vi "MeasureDistanceInImage.vi"() -> ()   [LabVIEW 2016]
uses:
  <vilib>/vision/NI_Vision_Development_Module.lvlib
  <vilib>/Utility/inputDevices.llb/mouseAcquire.vi
panel:
  in  "Pitch":dbl=75.5
  in  "Npixels":dbl=774.031
  in  "Nstrips":dbl=17.0
  out "Length (um)":dbl=1283.499968605464
  out "Conversion: \n1 pixel to um":dbl=1.6582023200621165
  out "Length (Pixels)":dbl=774.0309810671256
  out "Position 2":cluster{"X2 Value":dbl, "Y2 Value":dbl}={"X2 Value"=1797.893287435456, "Y2 Value"=1434.5183016105418}
  in  "Set Position 2":bool=TRUE
  out "Position 1":cluster{"X1 Value":dbl, "Y1 Value":dbl}={"X1 Value"=2571.9242685025815, "Y1 Value"=1434.5183016105418}
  in  "Set Position 1":bool=TRUE
  out "Analysis Image":T1(plugin-control)
  out "error out":errorcluster
  in  "X coord":dbl(slide)=1797.893287435456 max=2592.0 scale=0.0..3840.0
  in  "Y coord":dbl(slide)=1434.5183016105418 max=1944.0
  out "axis info":T2
  out "Array":T3(array[cluster])
  out "Intensity Histogram":T4(graph)={"Starting Value"=0.0, "Incremental Value"=1.0, "Histogram"=[197, 7029, 132892, 970999, 1117168, 291828, 56433, 20526, 12325, 9713, 7377, 5795, 5651, 5314, 3720, 2616, 1826, 1549, 1730, 1683, 1402, 1473, 1424, 1279, 1558, 1557, 1323, 1503, 1470, 1441, 1598, 1708, 1752, 2278, 2684, 3297, 5038, 7928, 11020, 15856, 18444, 15887, 15408, 15022, 16873, 25059, 31763, 32994, 39559, 44318, 45818, 56557, 59745, 55325, 61336, 58801, 49186, 48315, 39061, 30075, 29526, 26387, 22284, 22031, 20409, 17373, 17024, 16091, 13164, 13088, 12293, 10119, 10289, 9463, 7808, 8013, 7680, 6634, 7304, 7199, 6356, 6959, 6712, 5915, 6605, 6512, 5771, 6500, 6373, 6066, 6669, 6627, 6337, 6938, 7422, 7246, 8047, 8727, 8566, 10407, 11503, 11840, 14142, 16803, 17562, 22809, 26304, 27447, 33496, 37329, 37032, 44436, 46230, 42854, 47790, 47201, 42637, 44791, 43072, 37704, 38373, 35741, 30906, 30613, 28123, 23550, 24512, 22759, 19529, 19195, 18077, 15460, 16338, 15747, 13203, 13914, 13230, 11109, 11903, 10976, 8982, 9154, 8056, 6836, 6374, 5448, 4144, 3761, 2999, 2167, 1811, 1352, 905, 721, 529, 313, 215, 155, 87, 72, 41, 19, 11, 9, 3, 2, 1, 1, 0, 0, 0, 0, 0, 0, 0, 0, 0, 0, 0, 0, 0, 0, 0, 0, 0, 0, 0, 0, 0, 0, 0, 0, 0, 0, 0, 0, 0, 0, 0, 0, 0, 0, 0, 0, 0, 0, 0, 0, 0, 0, 0, 0, 0, 0, 0, 0, 0, 0, 0, 0, 0, 0, 0, 0, 0, 0, 0, 0, 0, 0, 0, 0, 0, 0, 0, 0, 0, 0, 0, 0, 0, 0, 0, 0, 0, 0, 0, 0, 0, 0, 0, 0, 0, 0, 0, 0]}
  in  "Path":path=path "E:/BNL/XYZstage+Camera_CollectedImages/02-06-2017/images/image_00_-53_-30_-1.png"
  # "Measure a distance in an image"
  # "Supply data for calibration calculation"
  # "readoutstrips_2 : 42, 956.746, 75.5\nSzoom1 : 16, 2323, 75.5"
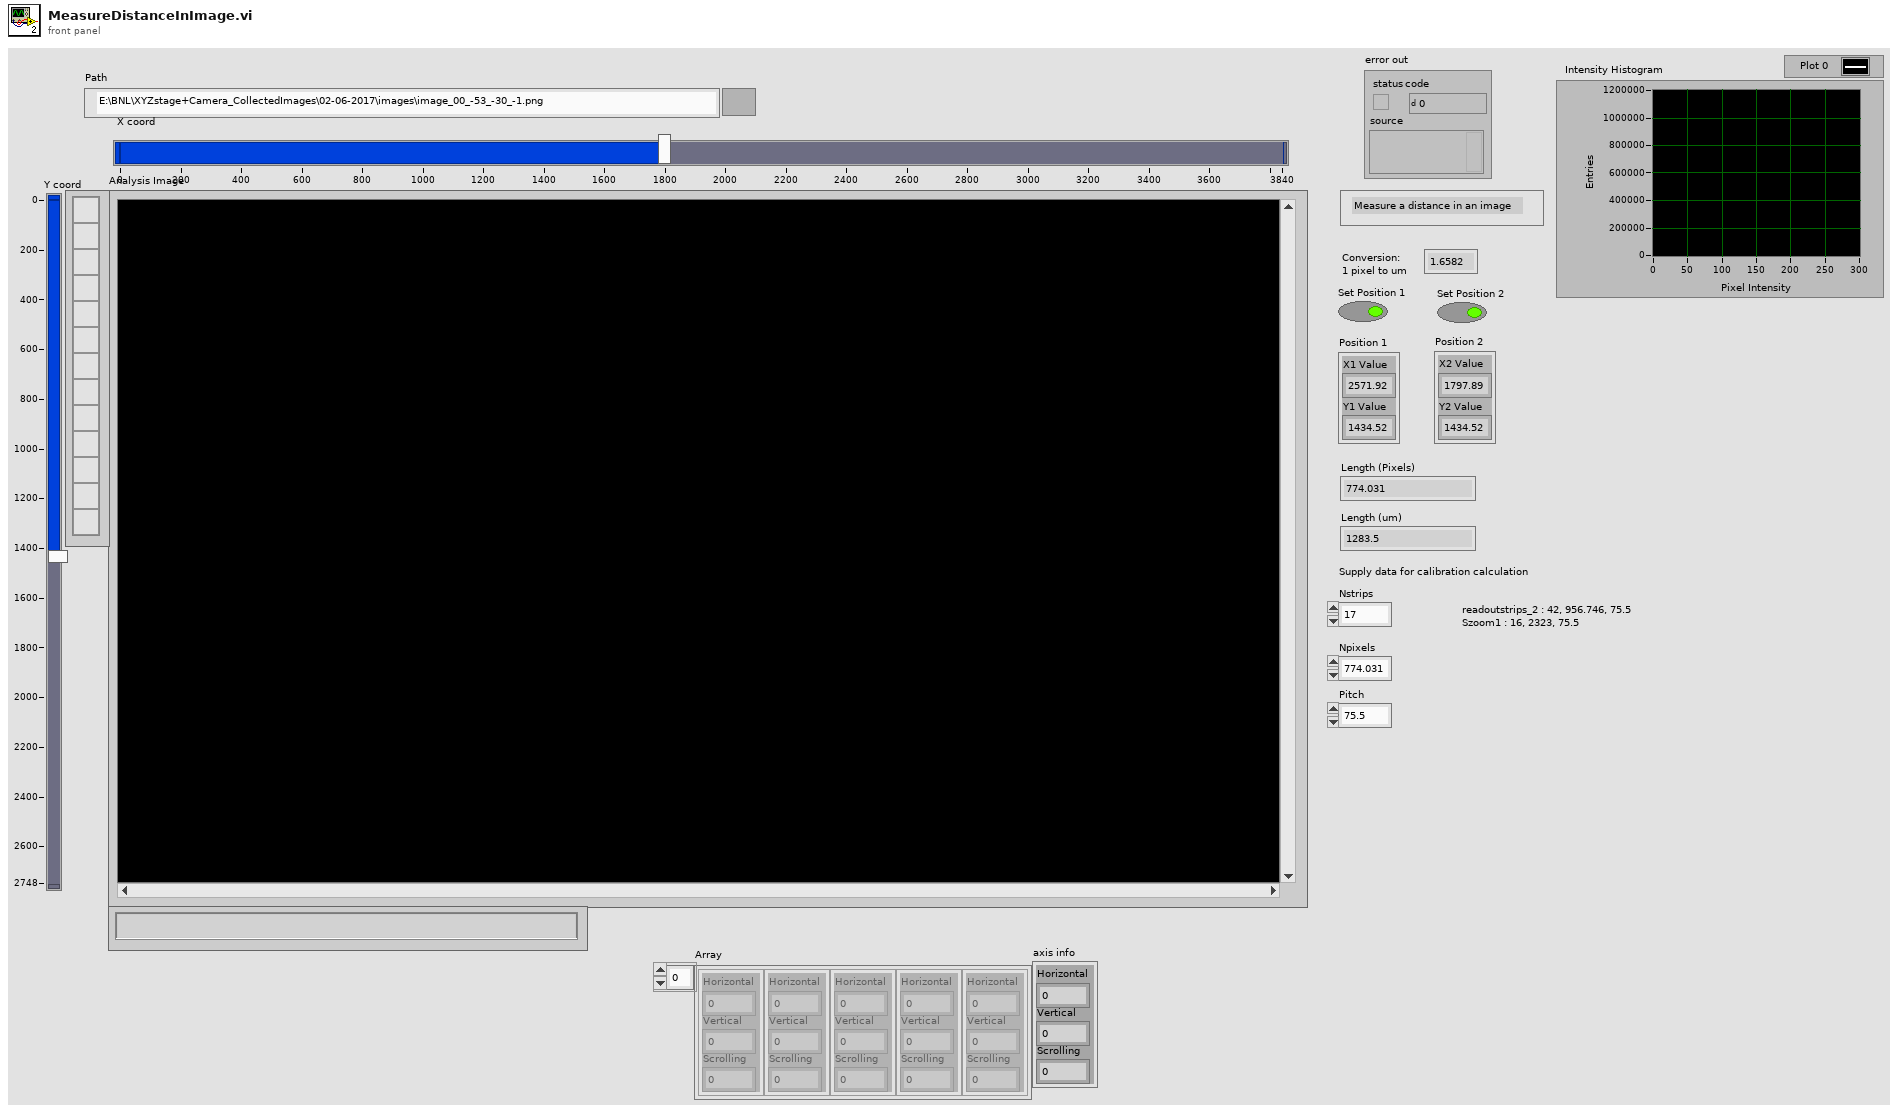
[diagram p1: front panel]
types:
  T1 = typedef "IMAQ Image.ctl" = refnum<image>
  T2 = cluster{"Horizontal":i32, "Vertical":i32, "Scrolling":i32}
  T3 = cluster{"Horizontal":i32, "Vertical":i32, "Scrolling":i32}[]
  T4 = cluster{"Starting Value":sgl, "Incremental Value":sgl, "Histogram":u32[]}
  T5 = cluster{"button 1":bool, "button 2":bool, "button 3":bool, "button 4":bool}
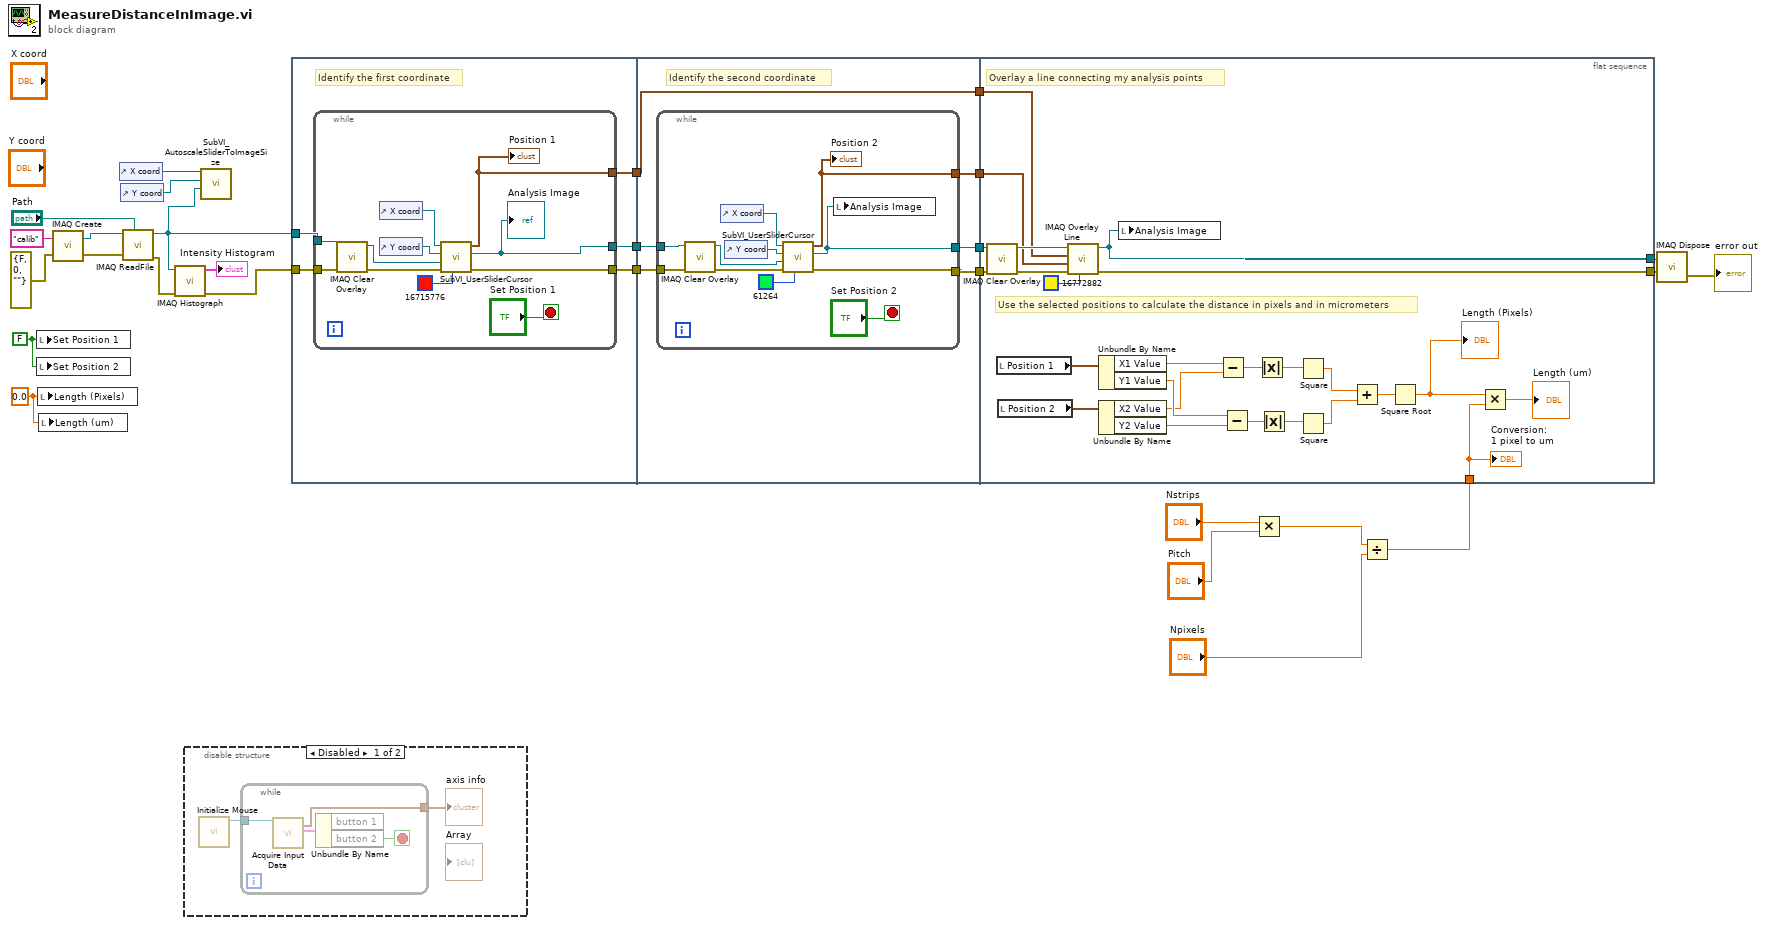
[diagram p0: block diagram]
diagram:
  w6 = 0.0 ("Length (Pixels)")
  w8 = FALSE ("Set Position 1")
  n1 = local write "Set Position 1"(w8) -> ()
  n2 = local write "Set Position 2"(w8) -> ()
  n3 = local write "Length (Pixels)"(w6) -> ()
  n4 = local write "Length (um)"(w6) -> ()
  n5 = call "IMAQ Create"("Image Name"="calib", "error in (no error)"=errorcluster {"status"=FALSE, "code"=0, "source"=""}) -> ("New Image"=w26:T1, "error out"=w25:errorcluster)  [unwired: 3 in]
  n6 = control-ref of="X coord"() -> (w19:refnum<vi>)
  n7 = control-ref of="Y coord"() -> (w18:refnum<vi>)
  n8 = call "IMAQ ReadFile"("File Path"="Path", "error in (no error)"=w25, "Image"=w26) -> ("error out"=w22:errorcluster, "Image Out"=w17:T1)  [unwired: 4 in, 3 out]
  n9 = call "IMAQ Histograph"("error in (no error)"=w22, "Image"=w17) -> ("error out"=w21:errorcluster, "Histogram Graph"=→"Intensity Histogram":T4)  [unwired: 6 in, 2 out]
  n10 = disable-structure shown="Disabled" {
    frame Disabled {
      n11 = call <vilib>:"Initialize Mouse.vi"() -> ("device ID"=w30:refnum<k1>)  [unwired: 10 in, 1 out]
      n12 = while {
        tunnel: w30 -> [w32]
        tunnel: [w31] -> w29
        stop <- w34 stop-if-true
        n13 = call-poly <vilib>:"Acquire Input Data.vi"("device ID"=w32) -> ("axis info"=w31:T2, "button info"=w33:T5)  [unwired: 15 in, 2 out]
        n14 = Unbundle By Name(w33) -> ("button 2"=w34:bool)  [unwired: 1 out]
      }
      "axis info" <- w29
    }
    frame Enabled {
    }
  }
  n15 = call "SubVI_AutoscaleSliderToImageSize.vi"("X slider refnum in"=w19, "Y slider refnum in"=w18, "Image RefNum"=w17) -> ()  [unwired: 7 in]
  n16 = flat-sequence {
    tunnel: w21 -> [w39]
    tunnel: w17 -> [w36]
    tunnel: [w38] -> w16
    tunnel: [w37] -> w15
    tunnel: [w35] -> w14
    tunnel: w16 -> [w55]
    tunnel: w15 -> [w54]
    tunnel: w14 -> [w53]
    tunnel: [w56] -> w13
    tunnel: [w53] -> w12
    tunnel: [w52] -> w11
    tunnel: [w51] -> w7
    tunnel: w13 -> [w85]
    tunnel: w12 -> [w84]
    tunnel: w11 -> [w92]
    tunnel: [w89] -> w10
    tunnel: [w88] -> w9
    tunnel: w7 -> [w86]
    tunnel: w1 -> [w68]
    frame #0 {
      # "Identify the first coordinate"
      n17 = while {
        tunnel: w36 -> [w50]
        tunnel: w39 -> [w49]
        tunnel: [w41] -> w38
        tunnel: [w42] -> w37
        tunnel: [w40] -> w35
        stop <- "Set Position 1" stop-if-true
        n18 = call "IMAQ Clear Overlay"("error in (no error)"=w49, "Image"=w50) -> ("error out"=w46:errorcluster, "Image Out"=w45:T1)  [unwired: 8 in]
        n19 = control-ref of="X coord"() -> (w43:refnum<vi>)
        n20 = control-ref of="Y coord"() -> (w44:refnum<vi>)
        n21 = call "SubVI_UserSliderCursor.vi"("Axes colour"=u32 16715776, "error in (no error)"=w46, "Image RefNum In"=w45, "Y slider refnum"=w44, "X slider refnum"=w43) -> ("error out"=w42:errorcluster, "Image Refnum out"=w41:T1, "Cross Point"=w40:cluster{"X coordinate":dbl, "Y coordinate":dbl})  [unwired: 4 in]
        "Analysis Image" <- w41
        "Position 1" <- w40
      }
    }
    frame #1 {
      # "Identify the second coordinate"
      n22 = while {
        tunnel: [w66] -> w52
        tunnel: [w57] -> w56
        tunnel: w55 -> [w63]
        tunnel: w54 -> [w62]
        tunnel: [w59] -> w51
        stop <- "Set Position 2" stop-if-true
        n23 = call "IMAQ Clear Overlay"("error in (no error)"=w62, "Image"=w63) -> ("error out"=w67:errorcluster, "Image Out"=w58:T1)  [unwired: 8 in]
        n24 = control-ref of="X coord"() -> (w60:refnum<vi>)
        n25 = control-ref of="Y coord"() -> (w61:refnum<vi>)
        n26 = call "SubVI_UserSliderCursor.vi"("Axes colour"=u32 61264, "error in (no error)"=w67, "Image RefNum In"=w58, "Y slider refnum"=w61, "X slider refnum"=w60) -> ("error out"=w66:errorcluster, "Image Refnum out"=w59:T1, "Cross Point"=w57:cluster{"X coordinate":dbl, "Y coordinate":dbl})  [unwired: 4 in]
        "Position 2" <- w57
        n27 = local write "Analysis Image"(w59) -> ()
      }
    }
    frame #2 {
      # "Use the selected positions to calculate the distance in pixels and in micrometers"
      # "Overlay a line connecting my analysis points"
      n28 = call "IMAQ Clear Overlay"("error in (no error)"=w92, "Image"=w86) -> ("error out"=w90:errorcluster, "Image Out"=w91:T1)  [unwired: 8 in]
      n29 = local read "Position 1"() -> (w72:cluster{"X1 Value":dbl, "Y1 Value":dbl})
      n30 = local read "Position 2"() -> (w73:cluster{"X2 Value":dbl, "Y2 Value":dbl})
      n31 = call "IMAQ Overlay Line"("Color"=u32 16772882, "error in (no error)"=w90, "End Point"=w85, "Start Point"=w84, "Image"=w91) -> ("error out"=w88:errorcluster, "Image Out"=w89:T1)  [unwired: 5 in]
      n32 = Unbundle By Name(w72) -> ("X1 Value"=w74:dbl, "Y1 Value"=w76:dbl)
      n33 = Unbundle By Name(w73) -> ("X2 Value"=w75:dbl, "Y2 Value"=w77:dbl)
      n34 = local write "Analysis Image"(w89) -> ()
      n35 = Subtract(x=w74, y=w75) -> (x-y=w78:dbl)
      n36 = Subtract(x=w76, y=w77) -> (x-y=w79:dbl)
      n37 = Absolute Value(x=w78) -> (abs(x)=w80:dbl)
      n38 = Absolute Value(x=w79) -> (abs(x)=w81:dbl)
      n39 = Square(x=w80) -> (x^2=w69:dbl)
      n40 = Square(x=w81) -> (x^2=w70:dbl)
      n41 = Add(x=w69, y=w70) -> (x+y=w71:dbl)
      n42 = Square Root(x=w71) -> (sqrt(x)=w82:dbl)
      "Length (Pixels)" <- w82
      n43 = Multiply(x=w82, y=w68) -> (x*y=→"Length (um)":dbl)
      "Conversion: \n1 pixel to um" <- w68
    }
  }
  n44 = Multiply(x="Nstrips", y="Pitch") -> (x*y=w2:dbl)
  n45 = Divide(x=w2, y="Npixels") -> (x/y=w1:dbl)
  n46 = call "IMAQ Dispose"("Image"=w10, "error in (no error)"=w9) -> ("error out"=→"error out":errorcluster)  [unwired: 4 in]
